vi "DAQ Set Analog Pin.vi"(8 "error in":errorcluster, 10 "Voltage":dbl format="%0.2f", 11 "task/channels in":refnum<k21>) -> (0 "error out":errorcluster, 2 "number of samples written per channel":u32, 3 "task out":refnum<k21>)   [LabVIEW 2021]
uses:
  <vilib>/DAQmx/write.llb/DAQmx Write (Analog DBL 1Chan 1Samp).vi
  <vilib>/DAQmx/miscellaneous.llb/DAQmx Fill In Error Info.vi
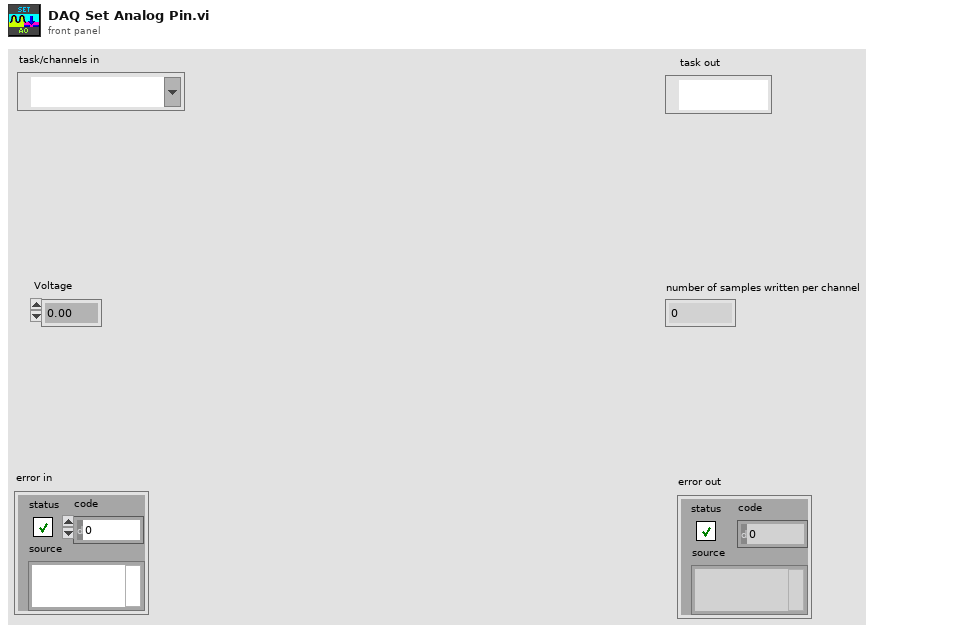
[diagram p1: front panel]
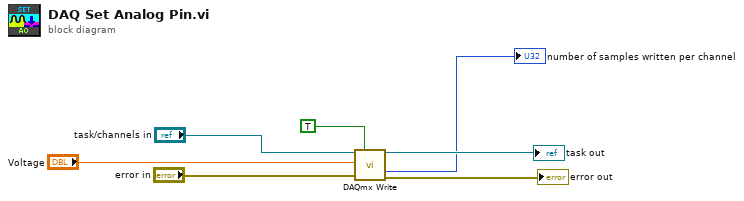
[diagram p0: block diagram]
diagram:
  n1 = call-poly <vilib>:"DAQmx Write.vi"("task/channels in"="task/channels in", "auto start"=TRUE, "data"="Voltage", "error in"="error in") -> ("task out"=→"task out":refnum<k21>, "number of samples written per channel"=→"number of samples written per channel":u32, "error out"=→"error out":errorcluster)  [unwired: 9 in]
